vi "글로벌 2.vi"() -> ()   [LabVIEW 2020]
panel:
  in  "클러스터":cluster{"배열":dbl[], "불리언":bool}
  out "불리언":bool
  out "숫자형 2":dbl
  in  "숫자형":dbl
  in  "정지":bool
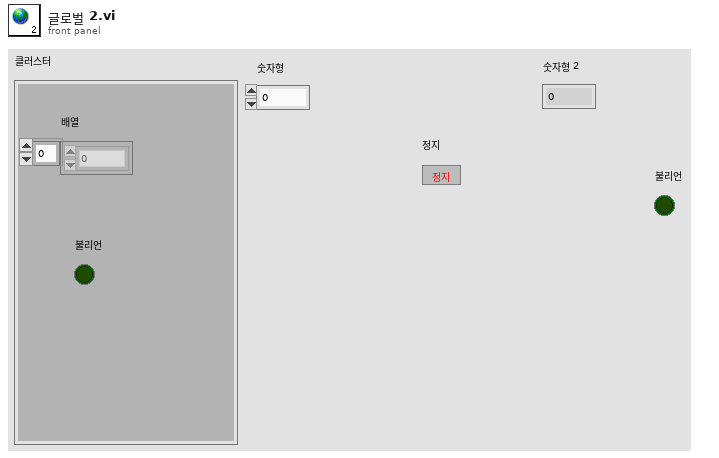
[diagram p1: front panel]
diagram:
